vi "全局 table.vi"() -> ()   [LabVIEW 2016]
panel:
  in  "table输入":string(combo)
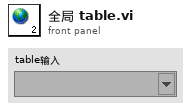
[diagram p1: front panel]
diagram:
